vi "Prozent 2 ppm.vi"(10 "Einheit":string(combo), 11 "Konzentration IST":dbl) -> (3 "Konzentration IST ppm":dbl)   [LabVIEW 2020, in "System Einstellungen V2.lvlib"]
uses:
  System Einstellungen V2.lvlib
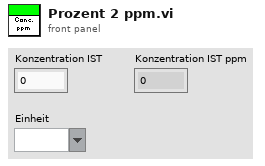
[diagram p1: front panel]
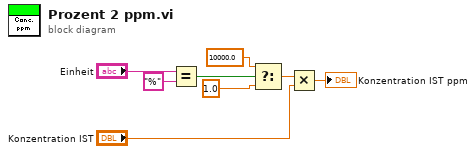
[diagram p0: block diagram]
diagram:
  n1 = Equal?(x="Einheit", y="%") -> (x = y?=w5:bool)
  n2 = Select(t=10000.0, s=w5, f=1.0) -> (s? t:f=w6:dbl)
  n3 = Multiply(x=w6, y="Konzentration IST") -> (x*y=→"Konzentration IST ppm":dbl)
